vi "ARGBImageGetChannelGreen.vi"(8 "error in (no error)":errorcluster, 10 "Greyscale Image Destination":refnum<data-value>, 11 "ARGB Image Source":refnum<data-value>) -> (0 "error out":errorcluster, 3 "Greyscale Image Destination (Duplicate)":refnum<data-value>)   [LabVIEW 2020, in "g_ar_toolkit.image.lvlib"]
uses:
  g_ar_toolkit.image.lvlib
  <vilib>/Utility/error.llb/Error Cluster From Error Code.vi
  ExtractOptions.ctl
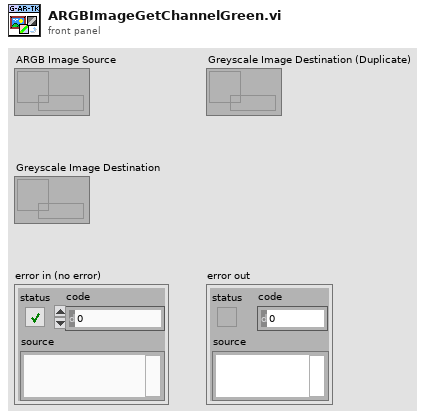
[diagram p1: front panel]
types:
  T1 = typedef "g_ar_toolkit.image.lvlib/ExtractOptions.ctl" = enum8{"Blue", "Green", "Red", "Alpha", "Greyscale"}
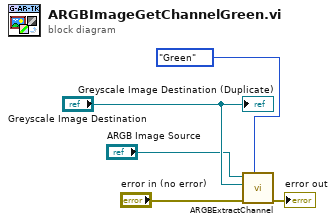
[diagram p0: block diagram]
diagram:
  n1 = call "ARGBExtractChannel.vi"("ExtractOperation"=ExtractOptions."Green" ("Extract_Operation"), "error in (no error)"="error in (no error)", "Greyscale Image Destination"="Greyscale Image Destination", "ARGB Image Source"="ARGB Image Source") -> ("error out"=→"error out":errorcluster)  [unwired: 7 in]
  "Greyscale Image Destination (Duplicate)" <- "Greyscale Image Destination"
